vi "hangok_mappa.vi"() -> (3 "*\\hang mapppa":path)   [LabVIEW 2014]
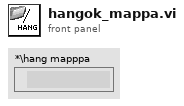
[diagram p1: front panel]
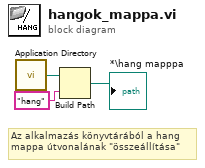
[diagram p0: block diagram]
diagram:
  # "Az alkalmazás könyvtárából a hang\nmappa útvonalának \"összeállítása\""
  n1 = call <vilib>:"Application Directory.vi"() -> ("Application Directory"=w2:path)
  n2 = Build Path(base path=w2, name or relative path="hang") -> (appended path=→"*\\hang mapppa":path)
